vi "Benchmark Convert String Type - Create Random Scalar Conversions.vi"(11 "channel count":i32) -> (3 "conversions":T1[](array[typedef]) {"converted descriptor"."buffer offset" format="%d bytes"; "unconverted descriptor"."buffer offset" format="%d bytes"})   [LabVIEW 2017]
uses:
  Classes/Buffer Converter/Type Conversion.ctl
  Classes/Buffer Converter/Channel Descriptor.ctl
  DSF Configuration API/Public/Controls/DSF Data Type.ctl
  DSF Core.lvlib
  Classes/Buffer/Buffer.lvclass
  Classes/Buffer Converter/Buffer Converter.lvclass
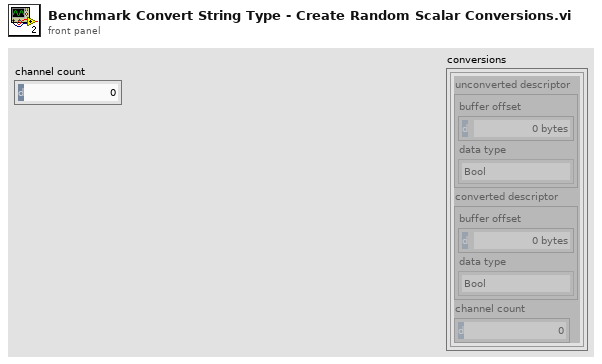
[diagram p1: front panel]
types:
  T1 = typedef "DSF Core.lvlib/Buffer Converter.lvclass/Type Conversion.ctl" = cluster{"unconverted descriptor":T2, "converted descriptor":T2, "channel count":u64}
  T2 = typedef "DSF Core.lvlib/Buffer.lvclass/Channel Descriptor.ctl" = cluster{"buffer offset":u64, "data type":T3}
  T3 = typedef "DSF Core.lvlib/DSF Data Type.ctl" = enum8{"Bool", "SGL", "DBL", "I8", "I16", "I32", "I64", "U8", "U16", "U32", "U64"}
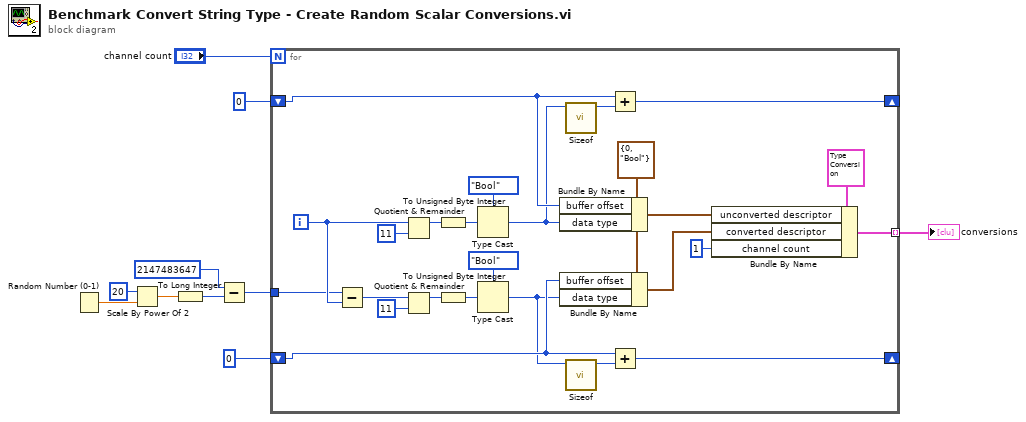
[diagram p0: block diagram]
diagram:
  n1 = Random Number (0-1)() -> (number: 0 to 1=w7:dbl)
  n2 = Scale By Power Of 2(n=i16 20, x=w7) -> (x*2^n=w5:dbl)
  n3 = To Long Integer(number=w5) -> (32bit integer=w3:i32)
  n4 = Subtract(x=2147483647, y=w3) -> (x-y=w2:i32)
  n5 = for {
    N: "channel count" -> [_]
    tunnel: [w33] -> w10 mode=indexing
    shift-right: [w31] -> _
    shift-left: u64 0 ("size in bytes") -> [w28]
    shift-right: [w25] -> _
    shift-left: u64 0 ("size in bytes") -> [w18]
    tunnel: w2 -> [w20]
    i -> [w21]
    w34 = T2 {"buffer offset"=0, "data type"=enum."Bool"} ("unconverted descriptor")
    n6 = Subtract(x=w20, y=w21) -> (x-y=w19:i32)
    n7 = Quotient & Remainder(x=w21, y=11) -> (x-y*floor(x/y)=w13:i32)  [unwired: 1 out]
    n8 = Quotient & Remainder(x=w19, y=11) -> (x-y*floor(x/y)=w23:i32)  [unwired: 1 out]
    n9 = To Unsigned Byte Integer(number=w13) -> (unsigned 8bit integer=w12:u8)
    n10 = To Unsigned Byte Integer(number=w23) -> (unsigned 8bit integer=w11:u8)
    n11 = Type Cast(type=DSF_Data_Type."Bool" ("data type"), x=w12) -> (*(type *) &x=w27:T3)
    n12 = Type Cast(type=DSF_Data_Type."Bool" ("data type"), x=w11) -> (*(type *) &x=w17:T3)
    n13 = Bundle By Name(cluster=w34, "buffer offset"=w28, "data type"=w27) -> (w16:T2)
    n14 = Bundle By Name(cluster=w34, "buffer offset"=w18, "data type"=w17) -> (w15:T2)
    n15 = call "Sizeof.vi"("data type"=w27) -> ("size in bytes"=w32:u64)  [unwired: 9 in, 1 out]
    n16 = call "Sizeof.vi"("data type"=w17) -> ("size in bytes"=w26:u64)  [unwired: 9 in, 1 out]
    n17 = Add(x=w28, y=w32) -> (x+y=w31:u64)
    n18 = Add(x=w18, y=w26) -> (x+y=w25:u64)
    n19 = Bundle By Name(cluster=T1 {"unconverted descriptor"={"buffer offset"=0, "data type"=enum."Bool"}, "converted descriptor"={"buffer offset"=0, "data type"=enum."Bool"}, "channel count"=0} ("conversion"), "unconverted descriptor"=w16, "converted descriptor"=w15, "channel count"=u64 1) -> (w33:T1)
  }
  "conversions" <- w10
